vi "Send UI Reference.vi"(8 "error in (no error)":errorcluster, 11 "Stage Controller in":refnum<class "Stage Controller.lvclass">) -> (0 "error out":errorcluster, 3 "Stage Controller out":refnum<class "Stage Controller.lvclass">)   [LabVIEW 2020, in "Stage.lvlib" / "Stage Controller.lvlib" / "Stage Controller.lvclass"]
uses:
  Stage Controller.lvclass
  C:/Program Files/National Instruments/LabVIEW 2020/vi.lib/ActorFramework/Actor/Actor.lvclass
  <vilib>/ActorFramework/Actor/Actor.lvclass/Actor.ctl
  Stage Controller.lvclass/Stage Controller.ctl
  Device/Device Messages/SendPanelUIReference Msg/SendPanelUIReference Msg.lvclass/SendPanelUIReference Msg.ctl
  <vilib>/ActorFramework/Message Enqueuer/Message Enqueuer.lvclass/Message Enqueuer.ctl
  <vilib>/ActorFramework/Message Enqueuer/Enqueue.vi
  Device/Device Messages/SendPanelUIReference Msg/SendPanelUIReference Msg.lvclass
  C:/Program Files/National Instruments/LabVIEW 2020/vi.lib/ActorFramework/Message/Message.lvclass
  <vilib>/ActorFramework/Message Priority Queue/Priority Enqueue.vi
  <vilib>/ActorFramework/Actor/Actor.lvclass
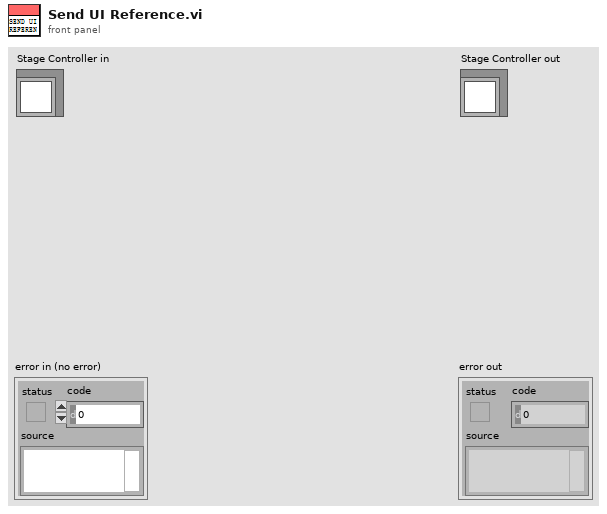
[diagram p1: front panel]
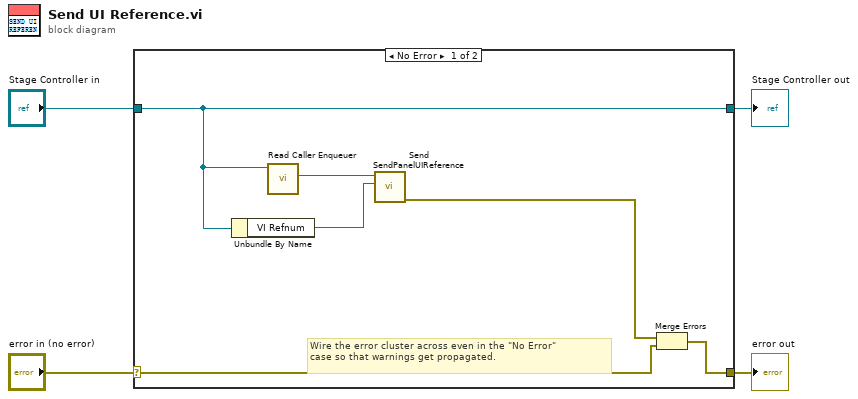
[diagram p0: block diagram]
diagram:
  n1 = case shown="No Error" "error in (no error)" {
    selector: "error in (no error)" -> [w10 w12]
    tunnel: [w9 w12] -> w3
    tunnel: [w6 w11] -> w1
    tunnel: "Stage Controller in" -> [w6 w11]
    frame No Error {
      # "Wire the error cluster across even in the \"No Error\"\ncase so that warnings get propagated."
      n2 = Unbundle By Name(w6) -> ("VI Refnum"=w5:refnum<vi>)
      n3 = call <vilib>:"Read Caller Enqueuer.vi"("Actor"=w6) -> ("Caller Enqueuer"=w8:refnum<class "Message Enqueuer.lvclass">)  [unwired: 10 in]
      n4 = call "Send SendPanelUIReference.vi"("VI Refnum"=w5, "Message Enqueuer"=w8) -> ("error out"=w7:errorcluster)  [unwired: 8 in, 1 out]
      n5 = Merge Errors(w7, w10) -> (w9:errorcluster)
    }
    frame Error {
    }
  }
  "error out" <- w3
  "Stage Controller out" <- w1
